vi "while_loop_time.vi"() -> ()   [LabVIEW 2017]
panel:
  in  "[ESC]":bool
  out "x-y 2":u32
  out "x-y":u32
  out "Numeric 2":i32
  out "Numeric":i32
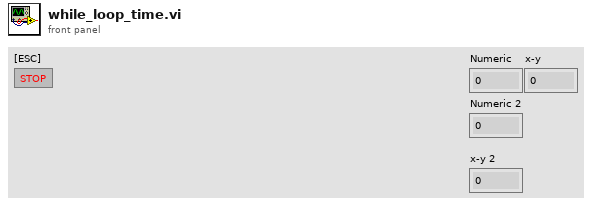
[diagram p1: front panel]
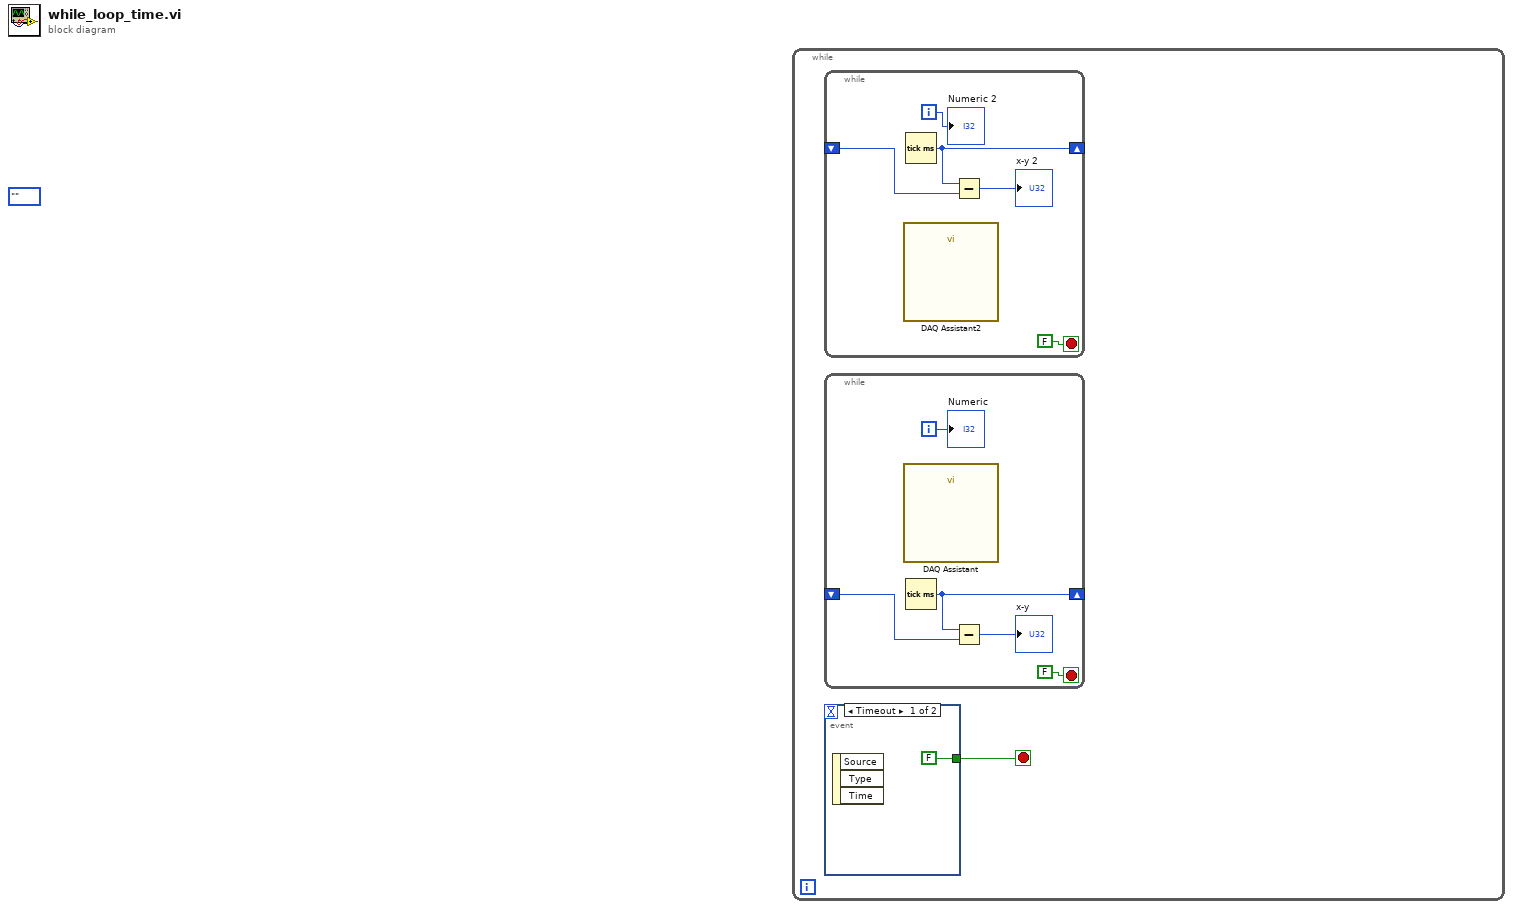
[diagram p0: block diagram]
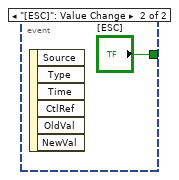
[diagram p2: hidden frame]
diagram:
  (unwired) enum16{""}.""
  n1 = while {
    stop <- w1 stop-if-true
    n2 = while {
      shift-right: [w2] -> _
      shift-left: _ -> [w3]
      i -> [w5]
      stop <- FALSE ("stop 2") stop-if-true
      n3 = call "DAQ Assistant2"() -> ()  [unwired: 16 in, 4 out]
      n4 = Tick Count (ms)() -> (millisecond timer value=w2:u32)
      n5 = Subtract(x=w2, y=w3) -> (x-y=→"x-y 2":u32)
      "Numeric 2" <- w5
    }
    n6 = while {
      shift-right: [w7] -> _
      shift-left: _ -> [w8]
      i -> [w10]
      stop <- FALSE ("stop") stop-if-true
      n7 = call "DAQ Assistant"() -> ()  [unwired: 16 in, 4 out]
      n8 = Tick Count (ms)() -> (millisecond timer value=w7:u32)
      n9 = Subtract(x=w7, y=w8) -> (x-y=→"x-y":u32)
      "Numeric" <- w10
    }
    n10 = event shown="[0] Timeout" {
      selector: _ -> [_ _]
      dyn-events: _ -> [_ _]
      timeout: _ -> [_ _]
      tunnel: [FALSE ("[ESC]") "[ESC]"] -> w1
      event Timeout {
        n11 = event-data() -> ()  [unwired: 1 in, 3 out]
      }
      event "[ESC]": Value Change {
        n12 = event-data() -> ()  [unwired: 1 in, 6 out]
      }
    }
  }
